vi "Prepare State Logic.vi"(8 "error in (no error)":errorcluster, 11 "CIFCorePlugin in":refnum<class "CIFCorePlugin.lvclass">) -> (0 "error out":errorcluster, 2 "Prepare State Logic":T1, 3 "CIFCorePlugin out":refnum<class "CIFCorePlugin.lvclass">)   [LabVIEW 2021, in "CIFCorePlugin.lvclass"]
uses:
  CIFCorePlugin.lvclass
  Typedef/Prepare State Logic.ctl
  CIFCorePlugin.lvclass/CIFCorePlugin.ctl
  CIFCoreCommon/Typedef/Plugin State.ctl
  CIFCoreCommon/CIFCoreCommon.lvlib
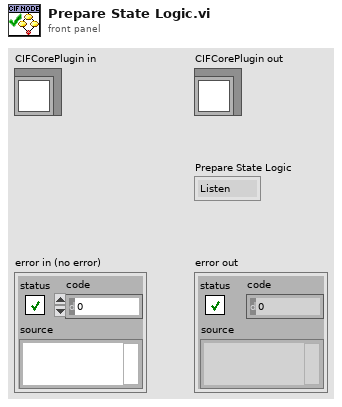
[diagram p1: front panel]
types:
  T1 = typedef "CIFCorePlugin.lvclass/Prepare State Logic.ctl" = enum16{"Listen", "Prepare", "Error", "Destroy"}
  T2 = typedef "CIFCorePlugin.lvclass/Energized States.ctl" = enum16{"Listen", "Prepare", "Execute", "Housekeep", "Cleanup", "Destroy"}
  T3 = typedef "CIFCoreCommon.lvlib/Plugin State.ctl" = enum32{"Null", "Creating", "Listening", "Running", "CleaningUp", "Destroying"}
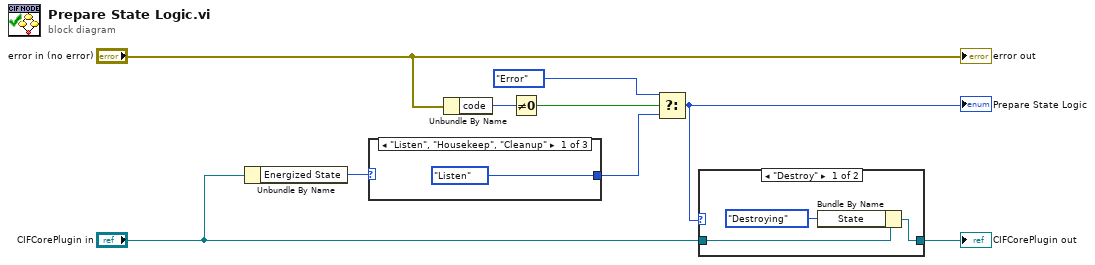
[diagram p0: block diagram]
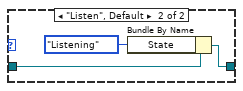
[diagram p2: hidden frame]
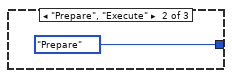
[diagram p3: hidden frame]
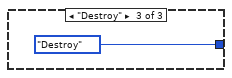
[diagram p4: hidden frame]
diagram:
  n1 = Unbundle By Name("CIFCorePlugin in") -> ("Energized State"=w5:T2)
  n2 = case shown="\"Listen\", \"Housekeep\", \"Cleanup\"" w5 {
    tunnel: [Prepare_State_Logic."Listen" ("Prepare State Logic") Prepare_State_Logic."Prepare" ("Prepare State Logic") Prepare_State_Logic."Destroy" ("Prepare State Logic")] -> w4
    frame "Listen", "Housekeep", "Cleanup" {
    }
    frame "Prepare", "Execute" {
    }
    frame "Destroy" {
    }
  }
  n3 = Unbundle By Name("error in (no error)") -> ("code"=w8:i32)
  n4 = Not Equal To 0?(x=w8) -> (x != 0?=w7:bool)
  n5 = Select(t=Prepare_State_Logic."Error" ("Prepare State Logic"), s=w7, f=w4) -> (s? t:f=w1:T1)
  "Prepare State Logic" <- w1
  n6 = case shown="\"Destroy\"" w1 {
    tunnel: "CIFCorePlugin in" -> [w14 w17]
    tunnel: [w13 w16] -> w2
    frame "Destroy" {
      n7 = Bundle By Name(cluster=w14, "State"=Plugin_State."Destroying" ("Status.State")) -> (w13:refnum<class "CIFCorePlugin.lvclass">)
    }
    frame "Listen", Default {
      n8 = Bundle By Name(cluster=w17, "State"=Plugin_State."Listening" ("Status.State")) -> (w16:refnum<class "CIFCorePlugin.lvclass">)
    }
  }
  "CIFCorePlugin out" <- w2
  "error out" <- "error in (no error)"
